vi "Destroy.vi"(8 "error in (no error)":errorcluster, 11 "QRCodeDetector in":refnum<class "QRDetector.lvclass">) -> (0 "error out":errorcluster)   [LabVIEW 2020, in "g_ar_toolkit.feature_detection.lvlib" / "QRDetector.lvclass"]
uses:
  QRDetector.lvclass
  QRDetector.lvclass/QRDetector.ctl
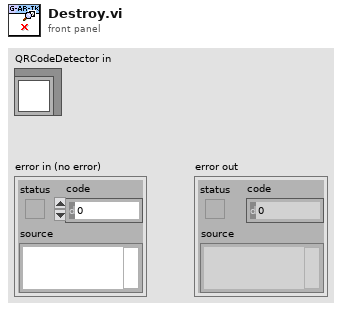
[diagram p1: front panel]
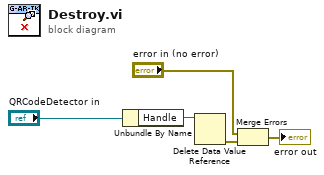
[diagram p0: block diagram]
diagram:
  n1 = Unbundle By Name("QRCodeDetector in") -> ("Handle"=w5:refnum<data-value>)
  n2 = Delete Data Value Reference(data value reference=w5) -> (error out=w2:errorcluster)  [unwired: 1 in, 1 out]
  n3 = Merge Errors("error in (no error)", w2) -> (→"error out":errorcluster)
